vi "FRAM_Write.vi"(8 "error in (no error)":errorcluster, 10 "Parameters":string, 11 "reference in":refnum<class "Test_Flux_Capacitor.lvclass">) -> (0 "error out":errorcluster, 2 "Result":bool, 3 "reference out":refnum<class "Test_Flux_Capacitor.lvclass">)   [LabVIEW 2022 SP3, in "Test_Flux_Capacitor.lvlib" / "Test_Flux_Capacitor.lvclass"]
uses:
  Test_Flux_Capacitor.lvclass
  <vilib>/numeric/Random Number (Range) U64.vi
  <vilib>/numeric/sub_Random U32.vi
  <vilib>/JDP Science/JSONtext/JSONtext.lvlib
panel:
  in  "Parameter_Type":cluster{"default":string}
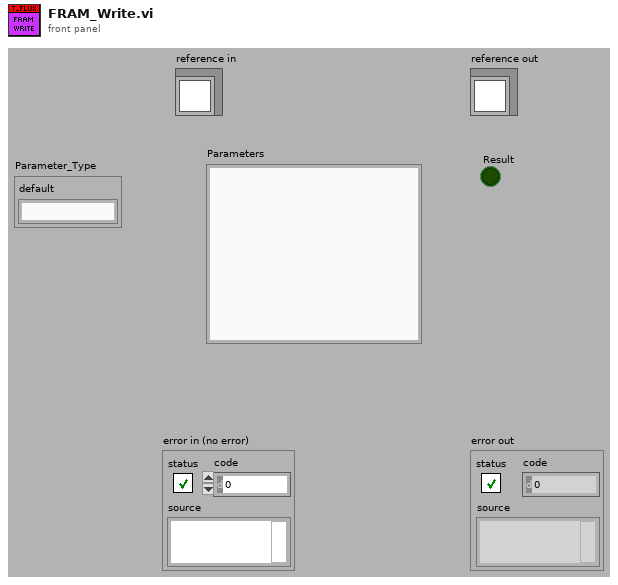
[diagram p1: front panel]
types:
  T1 = typedef "Test_Flux_Capacitor.lvlib/Test_Flux_Capacitor.lvclass/ObjectAttributes.ctl" = cluster{"Config":T2, "DMM":refnum<class "DMM_Keysight_34980A.lvclass">, "LCR":refnum<class "LCR_BK891.lvclass">, "PSU":refnum<class "PSU_Base.lvclass">, "Switch_Manager":refnum<class "SwitchBase.lvclass">, "FRAM":string, "Flux_Capacitor":refnum<class "Flux_Capacitor.lvclass">, "Frequency_Counter":refnum<class "Frequency_Counter_Base.lvclass">, "JTAG":refnum<class "JTAG_Base.lvclass">}
  T2 = typedef "Test_Flux_Capacitor.lvlib/Test_Flux_Capacitor.lvclass/Config.ctl" = cluster{"default":string}
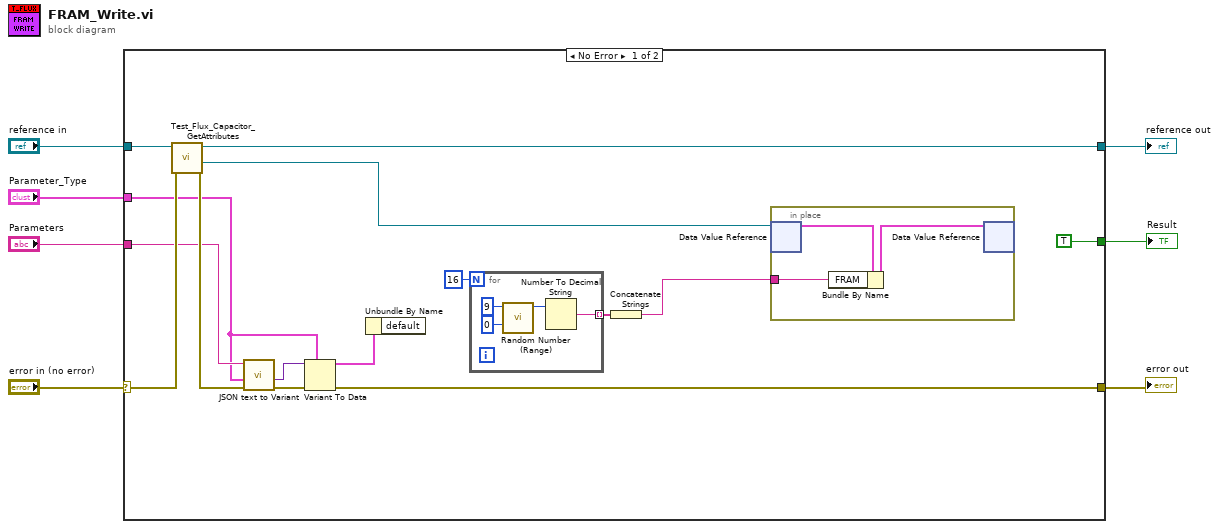
[diagram p0: block diagram]
diagram:
  n1 = case shown="No Error" "error in (no error)" {
    selector: "error in (no error)" -> [w22 w31]
    tunnel: [w8 w31] -> w6
    tunnel: [w18 w30] -> w4
    tunnel: "reference in" -> [w21 w30]
    tunnel: "Parameters" -> [w11 _]
    tunnel: "Parameter_Type" -> [w10 _]
    tunnel: [TRUE _] -> w1
    frame No Error {
      n2 = call "Test_Flux_Capacitor_GetAttributes.vi"("error in (no error)"=w22, "reference in"=w21) -> ("error out"=w13:errorcluster, "DataRef"=w15:refnum<data-value>, "reference out"=w18:refnum<class "Test_Flux_Capacitor.lvclass">)  [unwired: 6 in, 1 out]
      n3 = call <vilib>:"JSON text to Variant.vi"("error in (no error)"=w13, "Data Type"=w10, "JSON"=w11) -> ("error out"=w12:errorcluster, "Variant out"=w9:variant)  [unwired: 7 in]
      n4 = Variant To Data(error in=w12, type=w10, Variant=w9) -> (data=w20:cluster{"default":string}, error out=w8:errorcluster)
      n5 = Unbundle By Name(w20) -> ()  [unwired: 1 out]
      n6 = for {
        N: 16 -> [_]
        tunnel: [w26] -> w16 mode=indexing
        n7 = call-poly <vilib>:"Random Number (Range).vi"("lower bound (0)"=u64 0, "upper bound (100)"=u64 9) -> ("number"=w27:u64)  [unwired: 9 in]
        n8 = Number To Decimal String(number=w27) -> (decimal integer string=w26:string)  [unwired: 1 in]
      }
      n9 = Concatenate Strings(w16) -> (w14:string)
      n10 = in-place {
        in-place-border: w14 -> [w23]
        n11 = in-place-dvr #1(w15) -> (w25:T1)  [unwired: 1 out]
        n12 = Bundle By Name(cluster=w25, "FRAM"=w23) -> (w24:T1)
        n13 = in-place-dvr #1(w24) -> ()  [unwired: 2 out]
      }
    }
    frame Error {
    }
  }
  "Result" <- w1
  "error out" <- w6
  "reference out" <- w4
